vi "PQ Test List Tables.vi"(8 "error in (no error)":errorcluster, 10 "Connection String":string="user = llab_reader") -> (0 "error out":errorcluster)   [LabVIEW 2019, in "LV-Data.PGSQL.lvclass"]
uses:
  LV-Data.PGSQL.lvclass
  <vilib>/addons/_JKI Toolkits/Caraya/classes/Assert/Assert Not Error.vi
  <vilib>/addons/_JKI Toolkits/Caraya/classes/Assert/Assert.lvclass
  <vilib>/addons/_JKI Toolkits/Caraya/classes/Test/Test.lvclass
panel:
  out "delimited string":string
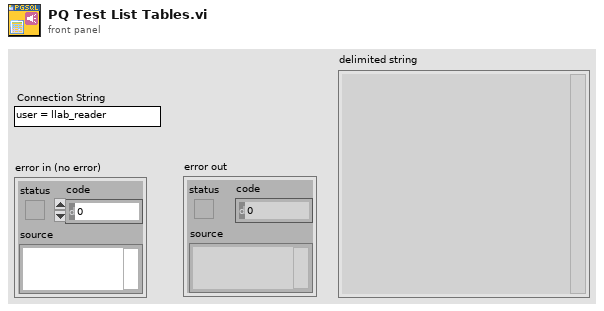
[diagram p1: front panel]
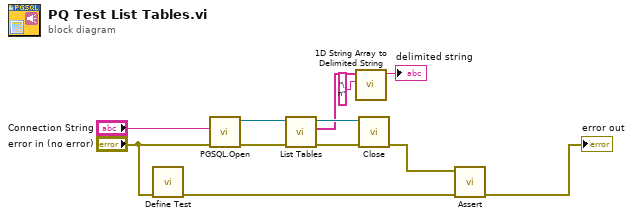
[diagram p0: block diagram]
diagram:
  n1 = call <vilib>:"Define Test.vi"("error in (no error)"="error in (no error)") -> ("error out"=w8:errorcluster)  [unwired: 9 in, 1 out]
  n2 = call "PGSQL.Open.vi"("error in (no error)"="error in (no error)", "Connection String"="Connection String") -> ("error out"=w6:errorcluster, "Data.PG out"=w7:refnum<class "LV-Data.PGSQL.lvclass">)  [unwired: 8 in]
  n3 = call "List Tables.vi"("error in (no error)"=w6, "Data.PG"=w7) -> ("error out"=w4:errorcluster, "Table Names"=w3:string[], "Data.PG"=w5:refnum<class "LV-Data.PGSQL.lvclass">)  [unwired: 6 in, 1 out]
  n4 = call <vilib>:"1D String Array to Delimited String.vi"("delimiter"="\n", "string array"=w3) -> ("delimited string"=→"delimited string":string)  [unwired: 9 in]
  n5 = call-dynamic "Close.vi"("error in (no error)"=w4, "Data.PG in"=w5) -> ("error out"=w11:errorcluster)  [unwired: 8 in, 1 out]
  n6 = call-poly <vilib>:"Assert.vi"("error in (no error)"=w8, "Not Error?"=w11) -> ("error out"=→"error out":errorcluster)  [unwired: 8 in, 1 out]
